vi "Get UI Details.vi"(8 "error in":errorcluster) -> (0 "error out":errorcluster, 3 "UserInterfaceDetails":T1)   [LabVIEW 2020, in "MeasurementTemplate_server.lvlib"]
uses:
  MeasurementTemplate_server.lvlib
  RPC Messages/ni_measurements_v1_UserInterfaceDetails.ctl
  Measurement UI.vi
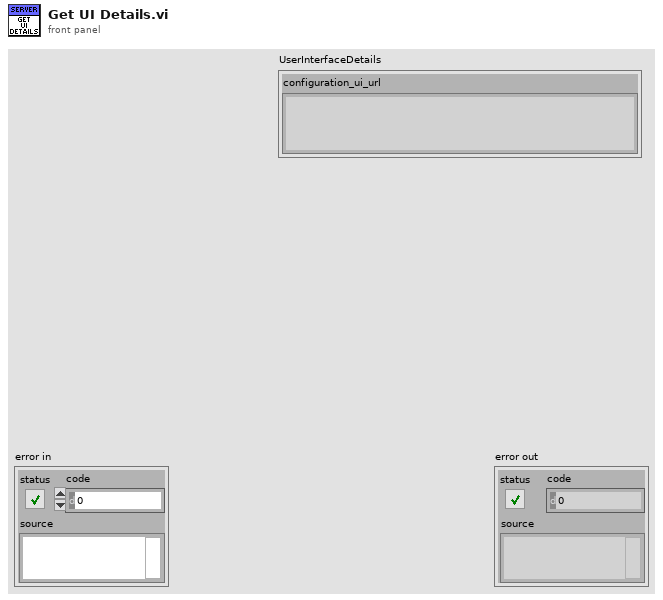
[diagram p1: front panel]
types:
  T1 = typedef "MeasurementTemplate_server.lvlib/ni_measurements_v1_UserInterfaceDetails.ctl" = cluster{"configuration_ui_url":string}
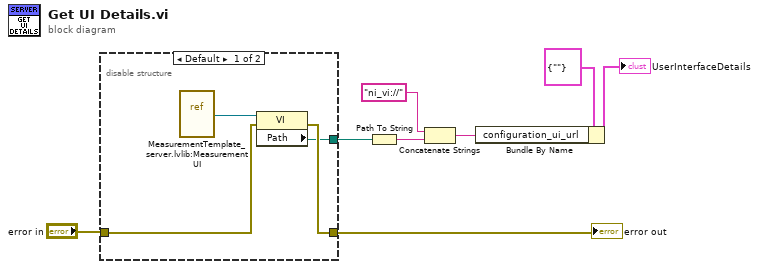
[diagram p0: block diagram]
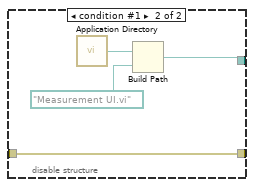
[diagram p2: hidden frame]
diagram:
  n1 = disable-structure shown="Default" {
    disable-tunnel: "error in" -> [w11 w13]
    disable-tunnel: [w10 w13] -> w1
    disable-tunnel: [w9 w14] -> w3
    frame condition #0 (active) {
      n2 = vi-ref "MeasurementTemplate_server.lvlib:Measurement UI.vi"() -> (w12:refnum<vi>)
      n3 = property class="VI"(reference=w12, error in=w11) -> (error out=w10:errorcluster, "Path"=w9:path)  [unwired: 1 out]
    }
    frame condition #1 {
      n4 = call <vilib>:"Application Directory.vi"() -> ("Application Directory"=w16:path)
      n5 = Build Path(base path=w16, name or relative path=path "Measurement UI.vi") -> (appended path=w14:path)
    }
  }
  "error out" <- w1
  n6 = Path To String(path=w3) -> (string=w6:string)
  n7 = Concatenate Strings("ni_vi://" ("string"), w6) -> (w5:string)
  n8 = Bundle By Name(cluster=T1 {"configuration_ui_url"=""} ("UserInterfaceDetails"), "configuration_ui_url"=w5) -> (→"UserInterfaceDetails":T1)
